vi "ScriptedStateMachine.vi"(8 "ErrorArray In":errorcluster[](array[cluster]), 9 "Data In":variant, 10 "Script":string[](array[string]), 11 "NISTBus In":refnum<class "NISTBus.lvclass">) -> (0 "ErrorArray Out":errorcluster[](array[cluster]), 1 "Data Out":variant, 3 "NISTBus Out":refnum<class "NISTBus.lvclass">)   [LabVIEW 2014, in "Bus.lvlib" / "NISTBus.lvclass"]
uses:
  NISTBus.lvclass
  Public/TypeDefs/clBusData.ctl
  FGenPlugins/MyPluginBaseClass/TypeDef/PluginParams.ctl
  NISTBus.lvclass/NISTBus.ctl
  WfrmGenerator/WfrmPlugins/EventPluginBaseClass/TypeDefs/dblEvtSignalArray.ctl
  WfrmGenerator/WfrmModule/PublicAPI/Arguments/Broadcasts/clErrorRpt.ctl
  <vilib>/Utility/error.llb/Error Cluster From Error Code.vi
  <vilib>/ErrorRing/Error Ring.xnode
  <userlib>/NIST/NISTErrorLib/NISTErrorLib.lvlib
  WfrmGenerator/WfrmModule/WfrmModule.lvlib
  WfrmGenerator/WfrmPlugins/EventPluginBaseClass/BaseWfrmPlugin.lvclass
  FGenPlugins/MyPluginBaseClass/NISTFGenPluginsBase.lvclass
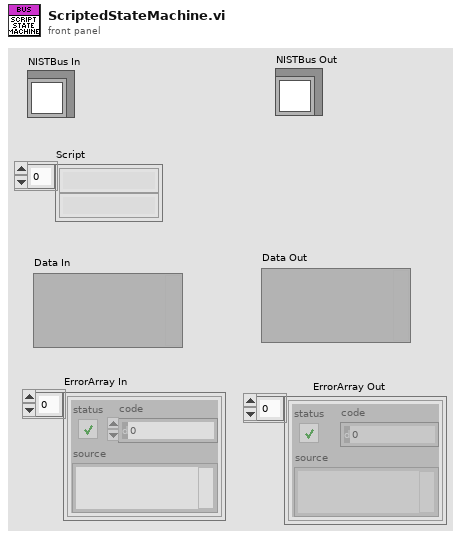
[diagram p1: front panel]
types:
  T1 = typedef "Bus.lvlib/NISTBus.lvclass/clBusData.ctl" = cluster{"BusNumber":u8, "NISTWfrmINIFilePath":path, "dblEventSignalArray":dbl[][], "NISTFGenPluginParams":T2}
  T2 = typedef "FGenPlugins.lvlib/NISTFGenPluginsBase.lvclass/PluginParams.ctl" = cluster{"Path to Plugin INI":path}
  T3 = typedef "WfrmModule.lvlib/clErrorRpt.ctl" = cluster{"error":errorcluster, "AdditionalInfo":string}
  T4 = typedef "TestFramework.lvlib/QueRef.ctl" = refnum<queue>
  T5 = typedef "WfrmModule.lvlib/clBroadcastEvents.ctl" = cluster{"DidInit":refnum<user-event>, "StatusUpdate":refnum<user-event>, "ErrorReport":refnum<user-event>, "DidStop":refnum<user-event>, "ReadEvtConfig":refnum<user-event>, "ReadTimeArray":refnum<user-event>, "ReadEvtParams":refnum<user-event>, "GetEvtReportArray":refnum<user-event>, "ReadPathToPlugin":refnum<user-event>, "GetEvtSignal":refnum<user-event>, "SendArbWfrm":refnum<user-event>}
  T6 = typedef "WfrmPlugins.lvlib/BaseWfrmPlugin.lvclass/dblEvtSignalArray.ctl" = dbl[][]
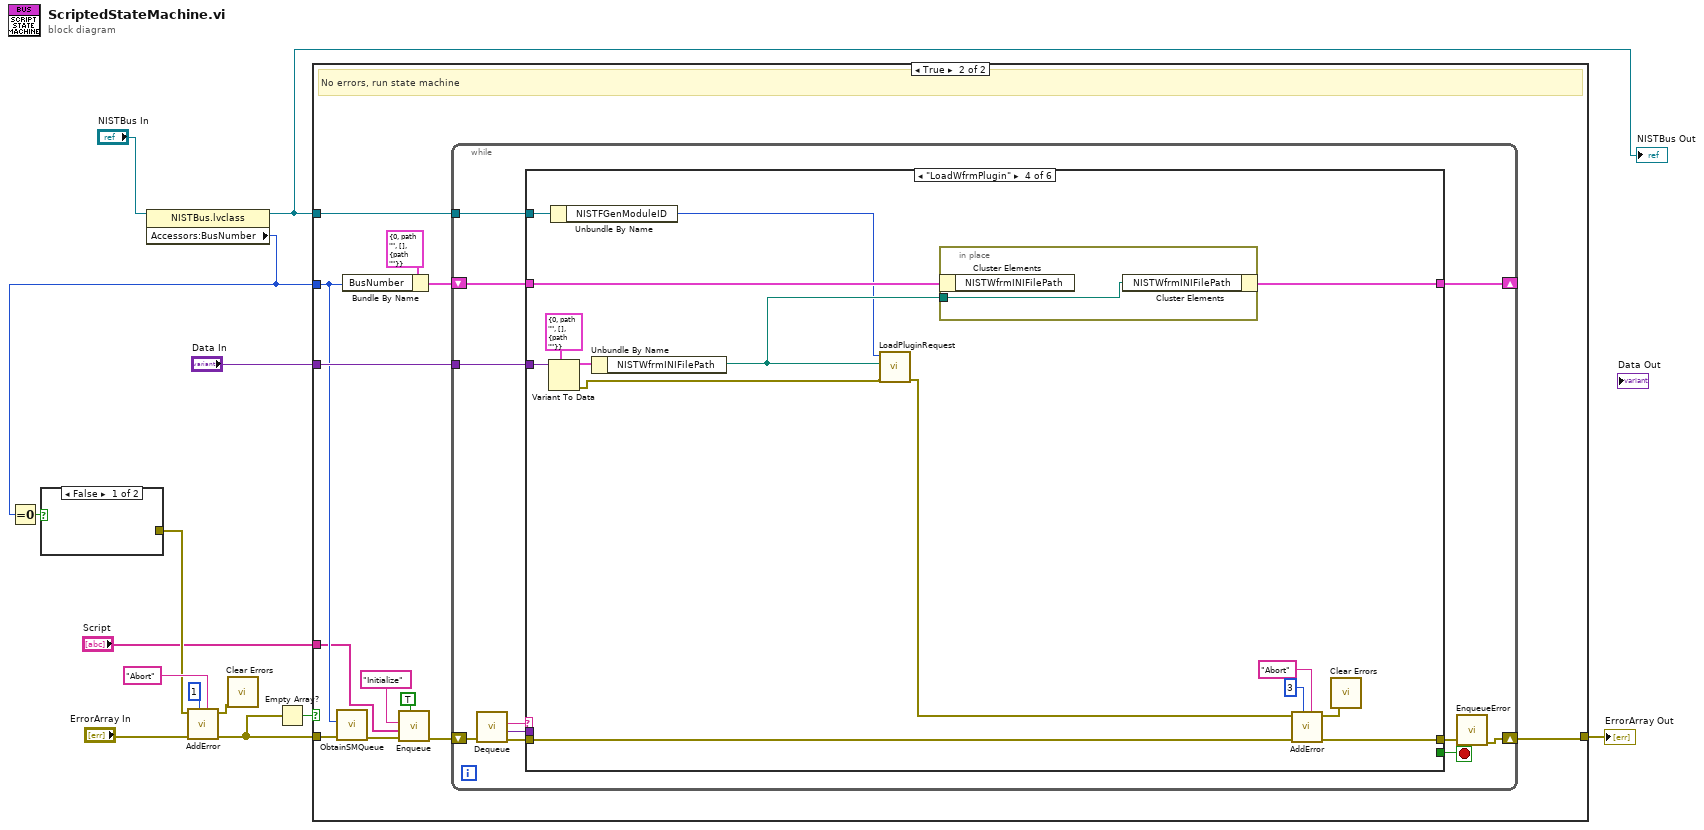
[diagram p0: block diagram]
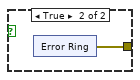
[diagram p2: hidden frame]
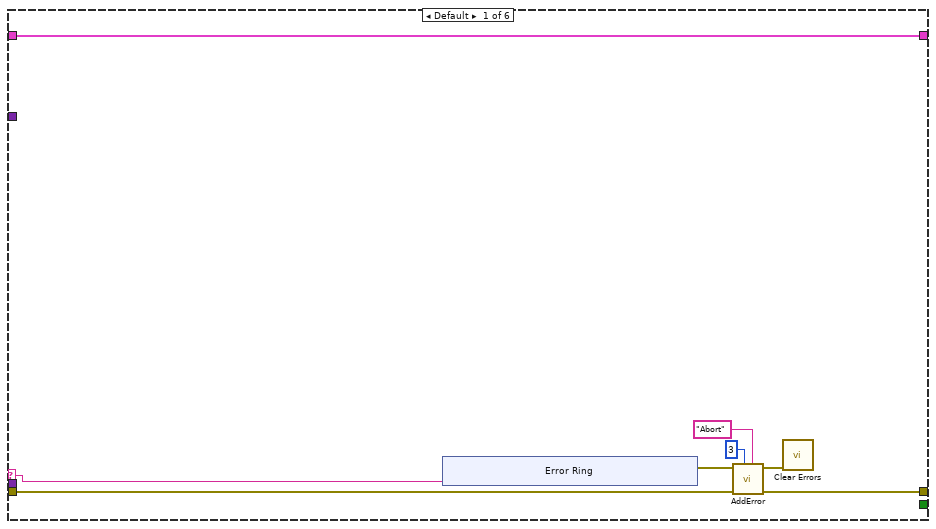
[diagram p4: hidden frame]
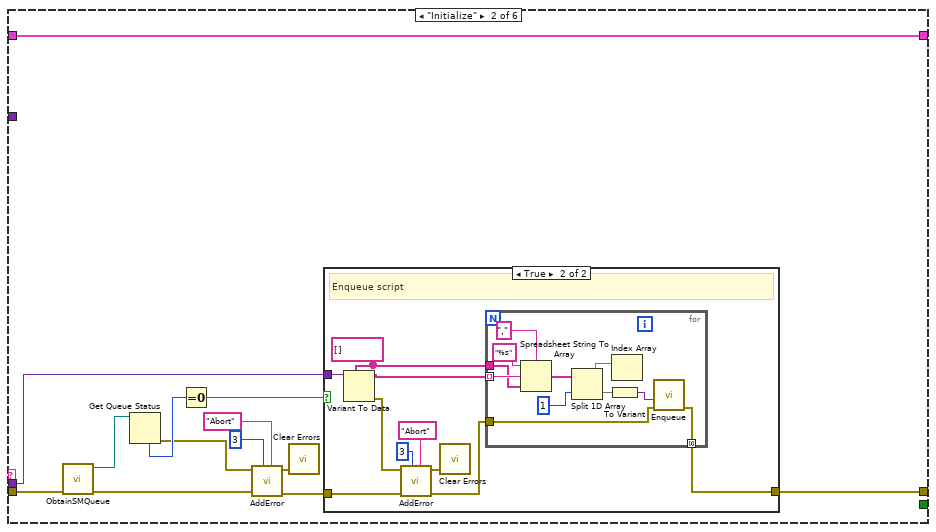
[diagram p5: hidden frame]
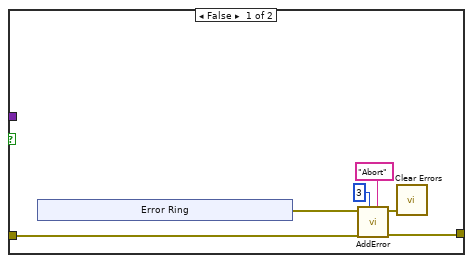
[diagram p6: hidden frame]
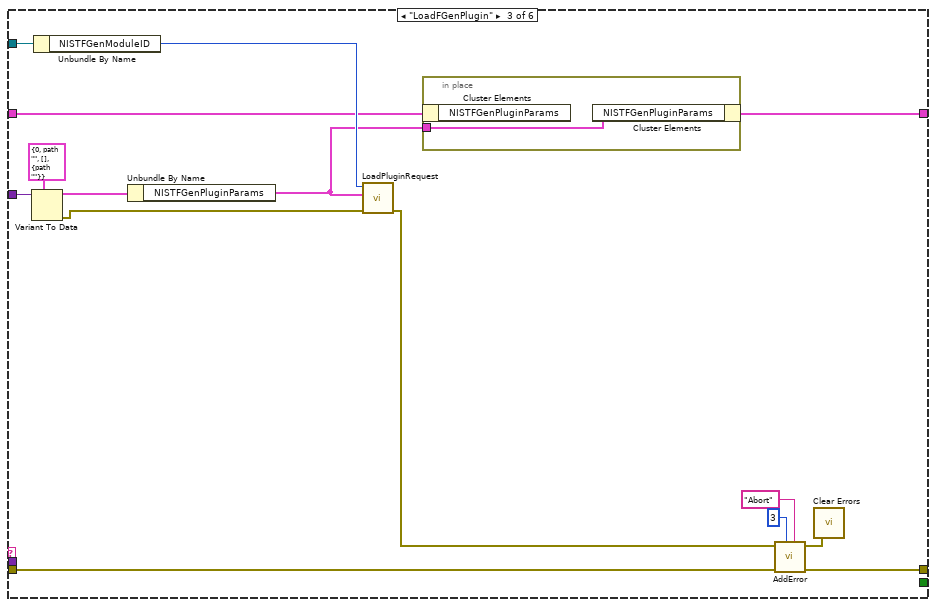
[diagram p7: hidden frame]
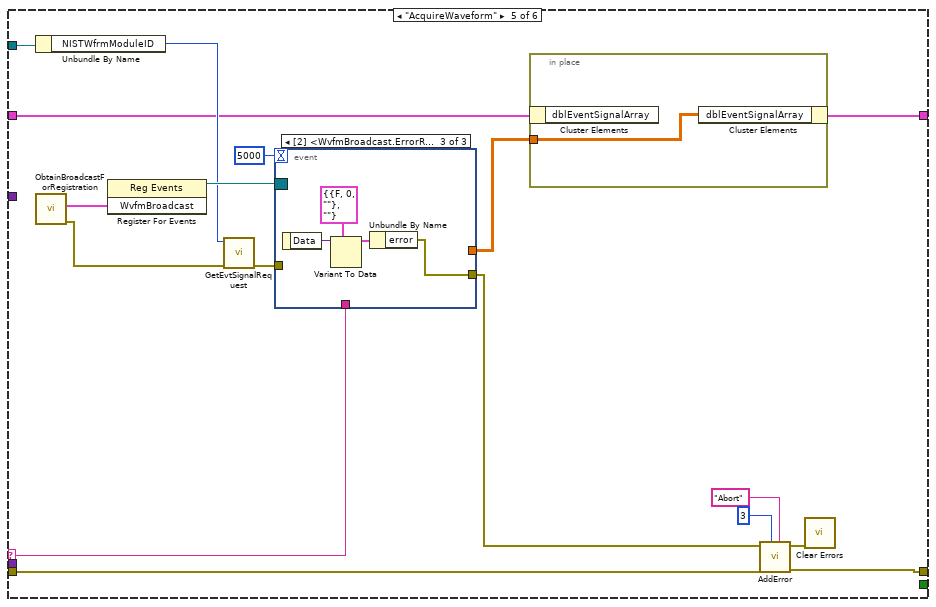
[diagram p8: hidden frame]
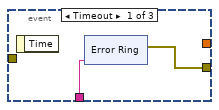
[diagram p9: hidden frame]
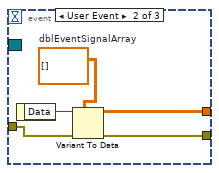
[diagram p10: hidden frame]
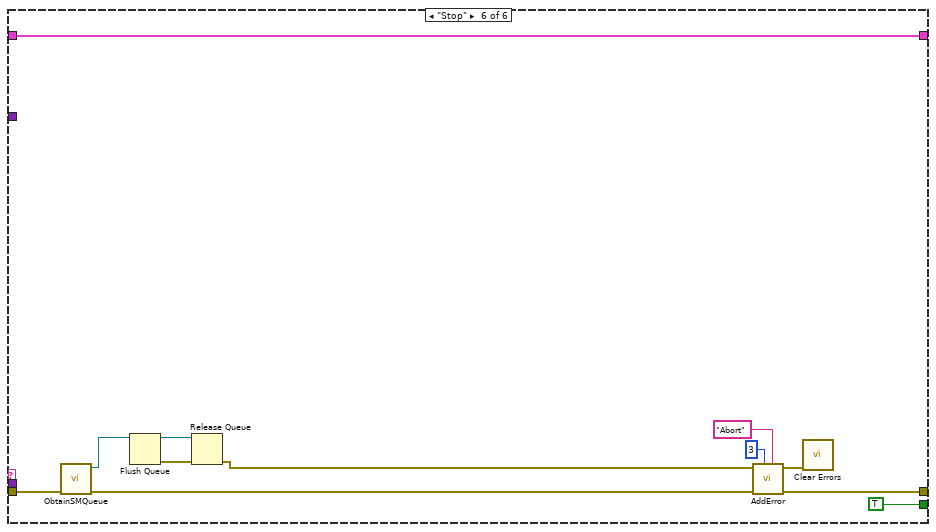
[diagram p11: hidden frame]
diagram:
  n1 = property class="NISTBus.lvclass"(reference="NISTBus In") -> (reference out=w1:refnum<class "NISTBus.lvclass">, "Accessors:BusNumber"=w6:u8)  [unwired: 1 in, 1 out]
  "NISTBus Out" <- w1
  n2 = Equal To 0?(x=w6) -> (x = 0?=w7:bool)
  n3 = case shown="False" w7 {
    tunnel: [_ w15] -> w5
    frame False {
    }
    frame True {
      n4 = xnode "Error Ring"() -> ("error out"=w15:errorcluster)
    }
  }
  n5 = call <userlib>:"AddError.vi"("Severity"="Abort" ("String"), "Priority"=u8 1, "ErrorArray"="ErrorArray In", "error in (no error)"=w5) -> ("ErrorArray"=w8:errorcluster[], "error out"=w10:errorcluster)  [unwired: 6 in]
  n6 = call <vilib>:"Clear Errors.vi"("error in (no error)"=w10) -> ()  [unwired: 5 in, 2 out]
  n7 = Empty Array?(array=w8) -> (empty?=w9:bool)
  n8 = case shown="True" w9 {
    tunnel: w8 -> [w17 w24]
    tunnel: w6 -> [_ w25]
    tunnel: "Script" -> [_ w21]
    tunnel: [w17 w18] -> w3
    tunnel: w1 -> [_ w27]
    tunnel: "Data In" -> [_ w26]
    frame False {
      # "Error entering state machine, do not run"
    }
    frame True {
      # "No errors, run state machine"
      n9 = call "ObtainSMQueue.vi"("ErrorArray In"=w24, "BusNumber"=w25) -> ("ErrorArray Out"=w20:errorcluster[])  [unwired: 8 in, 1 out]
      n10 = Bundle By Name(cluster=T1 {"BusNumber"=0, "NISTWfrmINIFilePath"=path "", "dblEventSignalArray"=[], "NISTFGenPluginParams"={"Path to Plugin INI"=path ""}} ("clBusData"), "BusNumber"=w25) -> (w28:T1)
      n11 = call "Enqueue.vi"("Priority (f)"=TRUE, "ErrorArray In"=w20, "Data"=w21, "Msg"="Initialize") -> ("ErrorArray Out"=w19:errorcluster[])  [unwired: 7 in]
      n12 = while {
        shift-right: [w31] -> _
        shift-left: w28 -> [w40]
        tunnel: w27 -> [w39]
        tunnel: w26 -> [w38]
        shift-right: [w32] -> w18
        shift-left: w19 -> [w37]
        stop <- w30 stop-if-true
        n13 = call "Dequeue.vi"("ErrorArray In"=w37) -> ("ErrorArray Out"=w36:errorcluster[], "Data"=w34:variant, "Msg"=w35:string)  [unwired: 8 in]
        n14 = case shown="\"LoadWfrmPlugin\"" w35 {
          selector: w35 -> [w43 _ _ _ w148 _]
          tunnel: w40 -> [w41 w56 w103 w122 w134 w169]
          tunnel: w39 -> [_ _ w105 w123 w140 _]
          tunnel: w38 -> [_ _ w115 w131 _ _]
          tunnel: w36 -> [w44 w68 w107 w124 w142 w179]
          tunnel: w34 -> [_ w58 _ _ _ _]
          tunnel: [w42 w59 w108 w125 w144 w172] -> w33
          tunnel: [w41 w56 w102 w121 w133 w169] -> w31
          tunnel: [_ _ _ _ _ TRUE] -> w30
          frame Default {
            n15 = xnode "Error Ring"("parameter 0"=w43) -> ("error out"=w46:errorcluster)
            n16 = call <userlib>:"AddError.vi"("Severity"="Abort" ("String"), "Priority"=u8 3, "ErrorArray"=w44, "error in (no error)"=w46) -> ("ErrorArray"=w42:errorcluster[], "error out"=w45:errorcluster)  [unwired: 6 in]
            n17 = call <vilib>:"Clear Errors.vi"("error in (no error)"=w45) -> ()  [unwired: 5 in, 2 out]
          }
          frame "Initialize" {
            n18 = call "ObtainSMQueue.vi"("ErrorArray In"=w68) -> ("ErrorArray Out"=w62:errorcluster[], "QueRef"=w61:T4)  [unwired: 9 in]
            n19 = Get Queue Status(queue=w61) -> (error out=w63:errorcluster, # elements in queue=w67:i32)  [unwired: 2 in, 6 out]
            n20 = Equal To 0?(x=w67) -> (x = 0?=w60:bool)
            n21 = call <userlib>:"AddError.vi"("Severity"="Abort" ("String"), "Priority"=u8 3, "ErrorArray"=w62, "error in (no error)"=w63) -> ("ErrorArray"=w57:errorcluster[], "error out"=w64:errorcluster)  [unwired: 6 in]
            n22 = call <vilib>:"Clear Errors.vi"("error in (no error)"=w64) -> ()  [unwired: 5 in, 2 out]
            n23 = case shown="True" w60 {
              tunnel: [w70 w89] -> w59
              tunnel: w58 -> [_ w84]
              tunnel: w57 -> [w69 w83]
              frame False {
                n24 = xnode "Error Ring"() -> ("error out"=w71:errorcluster)
                n25 = call <userlib>:"AddError.vi"("Severity"="Abort" ("String"), "Priority"=u8 3, "ErrorArray"=w69, "error in (no error)"=w71) -> ("ErrorArray"=w70:errorcluster[], "error out"=w72:errorcluster)  [unwired: 6 in]
                n26 = call <vilib>:"Clear Errors.vi"("error in (no error)"=w72) -> ()  [unwired: 5 in, 2 out]
              }
              frame True {
                w80 = string[] []
                # "Enqueue script"
                n27 = Variant To Data(type=w80, Variant=w84) -> (data=w81:string[], error out=w85:errorcluster)  [unwired: 1 in]
                n28 = call <userlib>:"AddError.vi"("Severity"="Abort" ("String"), "Priority"=u8 3, "ErrorArray"=w83, "error in (no error)"=w85) -> ("ErrorArray"=w82:errorcluster[], "error out"=w86:errorcluster)  [unwired: 6 in]
                n29 = call <vilib>:"Clear Errors.vi"("error in (no error)"=w86) -> ()  [unwired: 5 in, 2 out]
                n30 = for {
                  tunnel: [w94] -> w89 mode=concatenating
                  tunnel: w82 -> [w92]
                  tunnel: w81 -> [w91] mode=indexing
                  tunnel: w80 -> [w90]
                  n31 = Spreadsheet String To Array(delimiter (Tab)="," ("format string"), format string="%s", spreadsheet string=w91, array type (2D Dbl)=w90) -> (array=w98:string[])
                  n32 = Split 1D Array(array=w98, index=1) -> (first subarray=w95:string[], second subarray=w96:string[])
                  n33 = To Variant(anything=w96) -> (Variant=w93:variant)
                  n34 = Index Array(array=w95) -> ()  [unwired: 1 in, 1 out]
                  n35 = call "Enqueue.vi"("ErrorArray In"=w92, "Data"=w93) -> ("ErrorArray Out"=w94:errorcluster[])  [unwired: 9 in]
                }
              }
            }
          }
          frame "LoadFGenPlugin" {
            n36 = Variant To Data(type=T1 {"BusNumber"=0, "NISTWfrmINIFilePath"=path "", "dblEventSignalArray"=[], "NISTFGenPluginParams"={"Path to Plugin INI"=path ""}} ("clBusData"), Variant=w115) -> (data=w113:T1, error out=w112:errorcluster)  [unwired: 1 in]
            n37 = Unbundle By Name(w105) -> ("NISTFGenModuleID"=w104:i32)
            n38 = Unbundle By Name(w113) -> ("NISTFGenPluginParams"=w101:T2)
            n39 = call "LoadPluginRequest.vi"("error in (no error)"=w112, "PluginParams"=w101, "ModuleID"=w104) -> ("error out"=w106:errorcluster)  [unwired: 8 in]
            n40 = in-place {
              in-place-border: w101 -> [w116]
              n41 = in-place-cluster #1(w103) -> ()  [unwired: 1 out]
              n42 = in-place-cluster #1("NISTFGenPluginParams"=w116) -> (w102:T1)
            }
            n43 = call <userlib>:"AddError.vi"("Severity"="Abort" ("String"), "Priority"=u8 3, "ErrorArray"=w107, "error in (no error)"=w106) -> ("ErrorArray"=w108:errorcluster[], "error out"=w109:errorcluster)  [unwired: 6 in]
            n44 = call <vilib>:"Clear Errors.vi"("error in (no error)"=w109) -> ()  [unwired: 5 in, 2 out]
          }
          frame "LoadWfrmPlugin" {
            n45 = Variant To Data(type=T1 {"BusNumber"=0, "NISTWfrmINIFilePath"=path "", "dblEventSignalArray"=[], "NISTFGenPluginParams"={"Path to Plugin INI"=path ""}} ("clBusData"), Variant=w131) -> (data=w129:T1, error out=w118:errorcluster)  [unwired: 1 in]
            n46 = Unbundle By Name(w123) -> ("NISTFGenModuleID"=w119:i32)
            n47 = Unbundle By Name(w129) -> ("NISTWfrmINIFilePath"=w120:path)
            n48 = call "LoadPluginRequest.vi"("error in (no error)"=w118, "PathToPlugin"=w120, "ModuleID"=w119) -> ("error out"=w117:errorcluster)  [unwired: 8 in]
            n49 = in-place {
              in-place-border: w120 -> [w132]
              n50 = in-place-cluster #2(w122) -> ()  [unwired: 1 out]
              n51 = in-place-cluster #2("NISTWfrmINIFilePath"=w132) -> (w121:T1)
            }
            n52 = call <userlib>:"AddError.vi"("Severity"="Abort" ("String"), "Priority"=u8 3, "ErrorArray"=w124, "error in (no error)"=w117) -> ("ErrorArray"=w125:errorcluster[], "error out"=w126:errorcluster)  [unwired: 6 in]
            n53 = call <vilib>:"Clear Errors.vi"("error in (no error)"=w126) -> ()  [unwired: 5 in, 2 out]
          }
          frame "AcquireWaveform" {
            n54 = Unbundle By Name(w140) -> ("NISTWfrmModuleID"=w139:i32)
            n55 = call "ObtainBroadcastForRegistration.vi"() -> ("error out"=w137:errorcluster, "WvfmBroadcast"=w149:T5)  [unwired: 10 in]
            n56 = register-events(w149) -> (reference out=w141:refnum<event-registration>)  [unwired: 2 in, 1 out]
            n57 = call "GetEvtSignalRequest.vi"("error in (no error)"=w137, "ModuleID"=w139) -> ("error out"=w136:errorcluster)  [unwired: 9 in]
            n58 = event shown="[2] <WvfmBroadcast.ErrorReport>: User Event" {
              selector: w141 -> [_ _ _]
              dyn-events: _ -> [_ _ _]
              timeout: 5000 -> [_ _ _]
              tunnel: w148 -> [w152 _ _]
              tunnel: [w151 w162 w165] -> w143
              tunnel: w136 -> [_ w163 _]
              tunnel: [_ w160 _] -> w135
              event Timeout {
                n59 = event-data() -> ()  [unwired: 1 in, 1 out]
                n60 = xnode "Error Ring"("parameter 0"=w152) -> ("error out"=w151:errorcluster)
              }
              event User Event {
                w161 = T6 []  # dblEventSignalArray
                n61 = event-data() -> ("Data"=w164:variant)  [unwired: 1 in]
                n62 = Variant To Data(error in=w163, type=w161, Variant=w164) -> (data=w160:T6, error out=w162:errorcluster)
              }
              event User Event {
                n63 = event-data() -> ("Data"=w168:variant)  [unwired: 1 in]
                n64 = Variant To Data(type=T3 {"error"={"status"=FALSE, "code"=0, "source"=""}, "AdditionalInfo"=""} ("Cluster"), Variant=w168) -> (data=w166:T3)  [unwired: 1 in, 1 out]
                n65 = Unbundle By Name(w166) -> ("error"=w165:errorcluster)
              }
            }
            n66 = in-place {
              in-place-border: w135 -> [w150]
              n67 = in-place-cluster #3(w134) -> ()  [unwired: 1 out]
              n68 = in-place-cluster #3("dblEventSignalArray"=w150) -> (w133:T1)
            }
            n69 = call <userlib>:"AddError.vi"("Severity"="Abort" ("String"), "Priority"=u8 3, "ErrorArray"=w142, "error in (no error)"=w143) -> ("ErrorArray"=w144:errorcluster[], "error out"=w145:errorcluster)  [unwired: 6 in]
            n70 = call <vilib>:"Clear Errors.vi"("error in (no error)"=w145) -> ()  [unwired: 5 in, 2 out]
          }
          frame "Stop" {
            n71 = call "ObtainSMQueue.vi"("ErrorArray In"=w179) -> ("ErrorArray Out"=w171:errorcluster[], "QueRef"=w178:T4)  [unwired: 9 in]
            n72 = Flush Queue(queue=w178) -> (queue out=w177:T4, error out=w176:errorcluster)  [unwired: 1 in, 1 out]
            n73 = Release Queue(queue=w177, error in (no error)=w176) -> (error out=w170:errorcluster)  [unwired: 1 in, 2 out]
            n74 = call <userlib>:"AddError.vi"("Severity"="Abort" ("String"), "Priority"=u8 3, "ErrorArray"=w171, "error in (no error)"=w170) -> ("ErrorArray"=w172:errorcluster[], "error out"=w173:errorcluster)  [unwired: 6 in]
            n75 = call <vilib>:"Clear Errors.vi"("error in (no error)"=w173) -> ()  [unwired: 5 in, 2 out]
          }
        }
        n76 = call "EnqueueError.vi"("ErrorArray In"=w33) -> ("ErrorArray Out"=w32:errorcluster[])  [unwired: 10 in]
      }
    }
  }
  "ErrorArray Out" <- w3
